vi "PMBus Group Cmd.vi"(5 "PEC":u8, 6 "CmdNum":u8, 7 "pGroupCmdData":string, 8 "error in (no error)":errorcluster, 9 "PMBusIndex":i32, 10 "DevIndex":i32, 11 "DevType":i32) -> (0 "error out":errorcluster, 2 "function return":i32, 3 "pGroupCmdData out":string)   [LabVIEW 2012, in "ControlPMBus.lvlib"]
doc: "int WINAPI PMBus_GroupCmd(int DevType,int DevIndex,int PMBusIndex,unsigned char *pGroupCmdData,unsigned char CmdNum,unsigned char PEC);"
uses:
  ControlPMBus.lvlib
  Ginkgo_Driver.dll
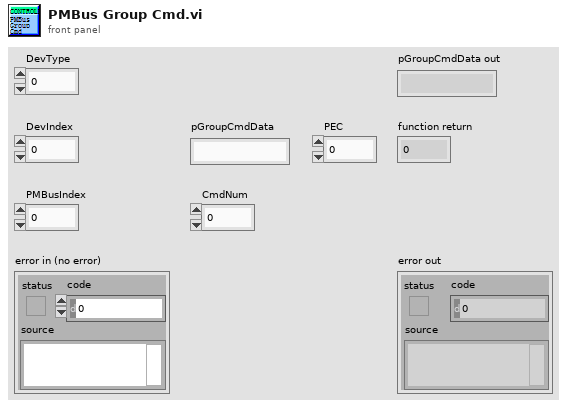
[diagram p1: front panel]
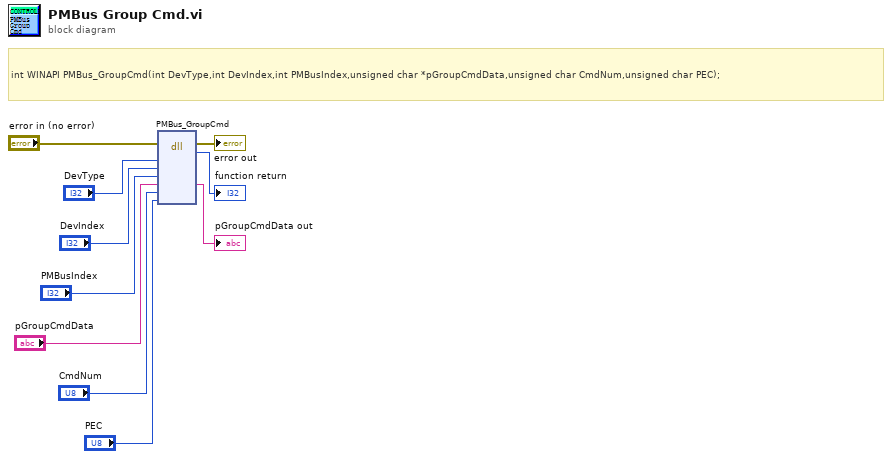
[diagram p0: block diagram]
diagram:
  # "int WINAPI PMBus_GroupCmd(int DevType,int DevIndex,int PMBusIndex,unsigned char *pGroupCmdData,unsigned char CmdNum,unsigned char PEC);"
  n1 = dll-call lib="E:/Project/vt_ginkgo/truck/Ginkgo Driver/vs2010/Ginkgo_USB-I2C_API_v2.0.3.0/lib/labview_64bit/ControlPMBus/Ginkgo_Driver.*" fn="PMBus_GroupCmd"(error in="error in (no error)", "DevType"="DevType", "DevIndex"="DevIndex", "PMBusIndex"="PMBusIndex", "pGroupCmdData"="pGroupCmdData", "CmdNum"="CmdNum", "PEC"="PEC") -> (error out=→"error out":errorcluster, →"function return":i32, "pGroupCmdData"=→"pGroupCmdData out":string)  [unwired: 7 in, 1 out]
